vi "UI_Users_Manage.vi"() -> ()   [LabVIEW 2014]
panel:
  in  "选项卡控件":enum32{"添加用户", "删除用户"}(tab)
  in  "身份":u16(ring) items=["普通用户", "管理员"]
  in  "添加":bool
  in  "密码":string
  in  "添加用户名":string caption="用户名"
  in  "删除":bool
  in  "删除用户名":string caption="用户名"
  in  "导出excel":bool
  out "用户信息":string[][](table)
  in  "退出":bool
  # "用户管理"
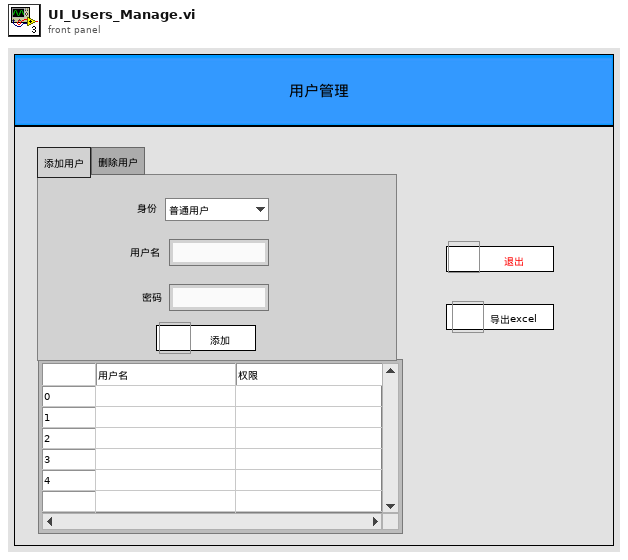
[diagram p1: front panel]
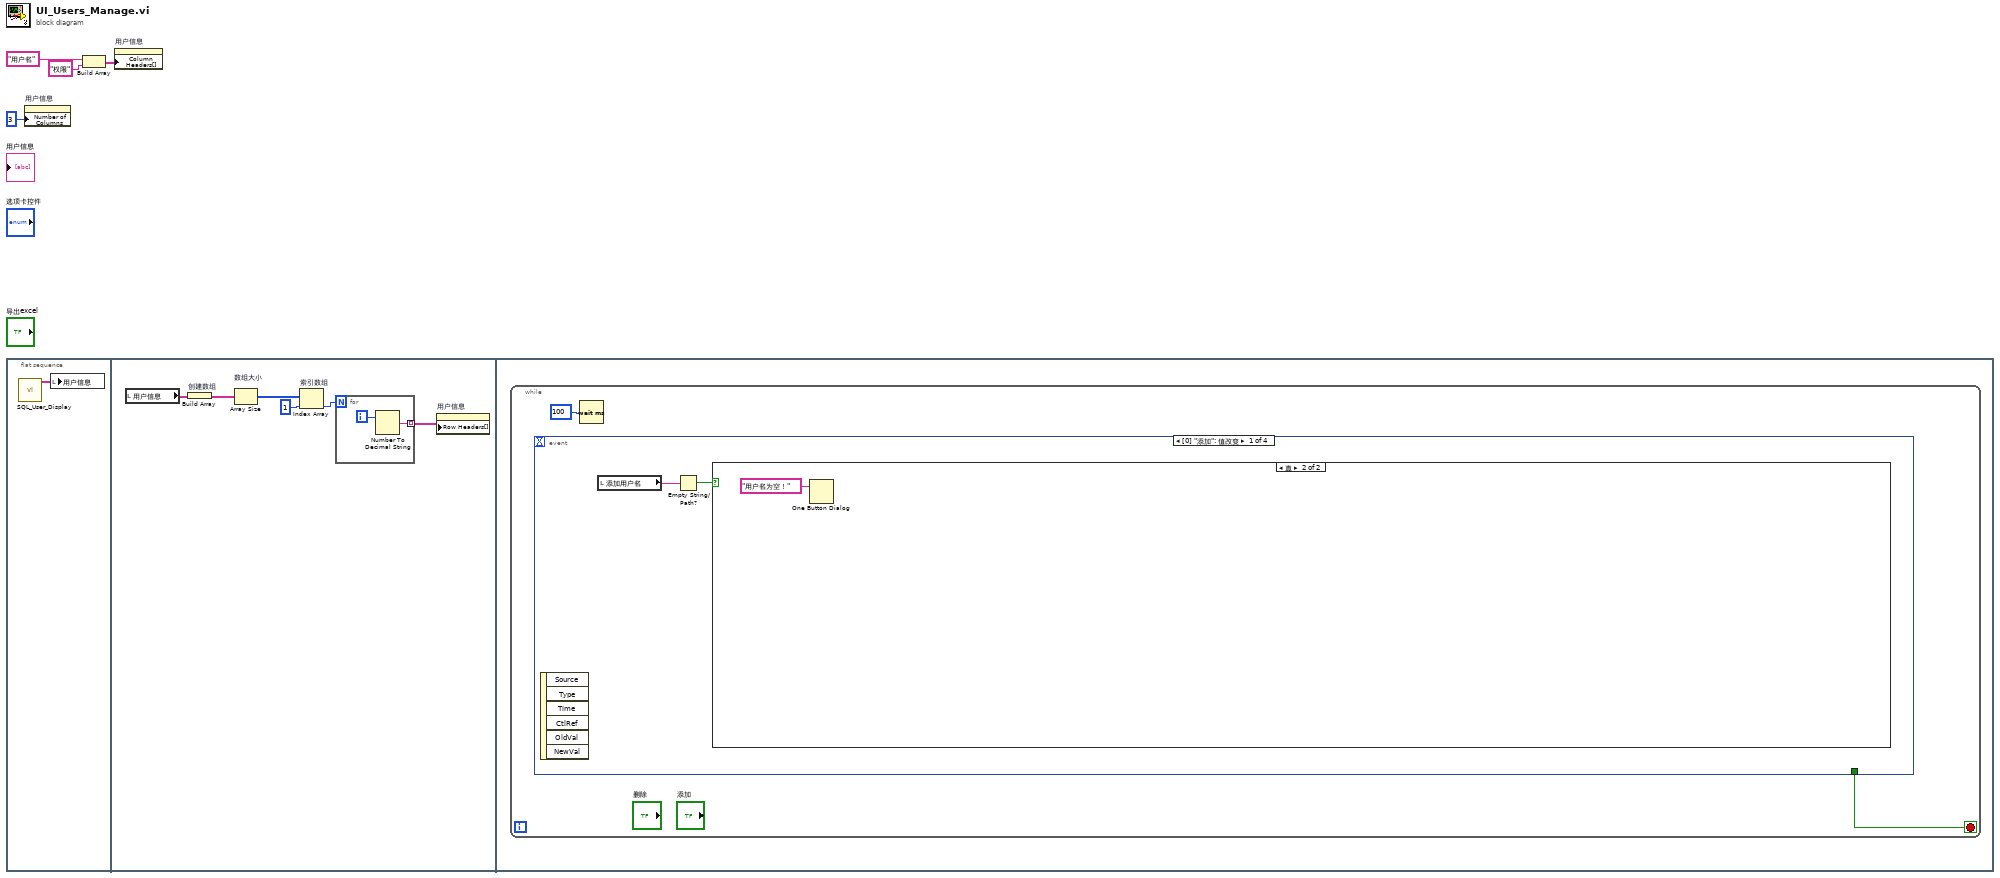
[diagram p0: block diagram]
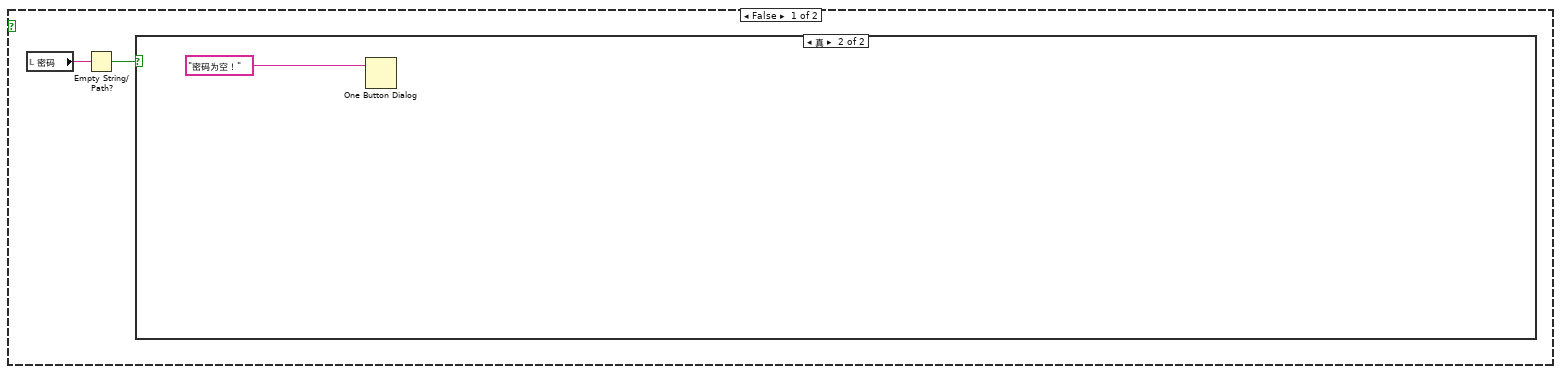
[diagram p2: hidden frame]
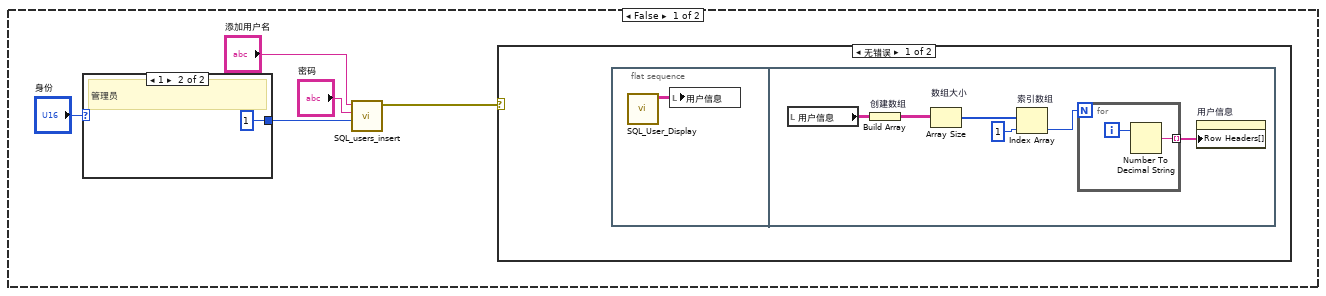
[diagram p3: hidden frame]
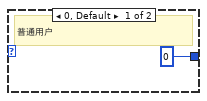
[diagram p5: hidden frame]
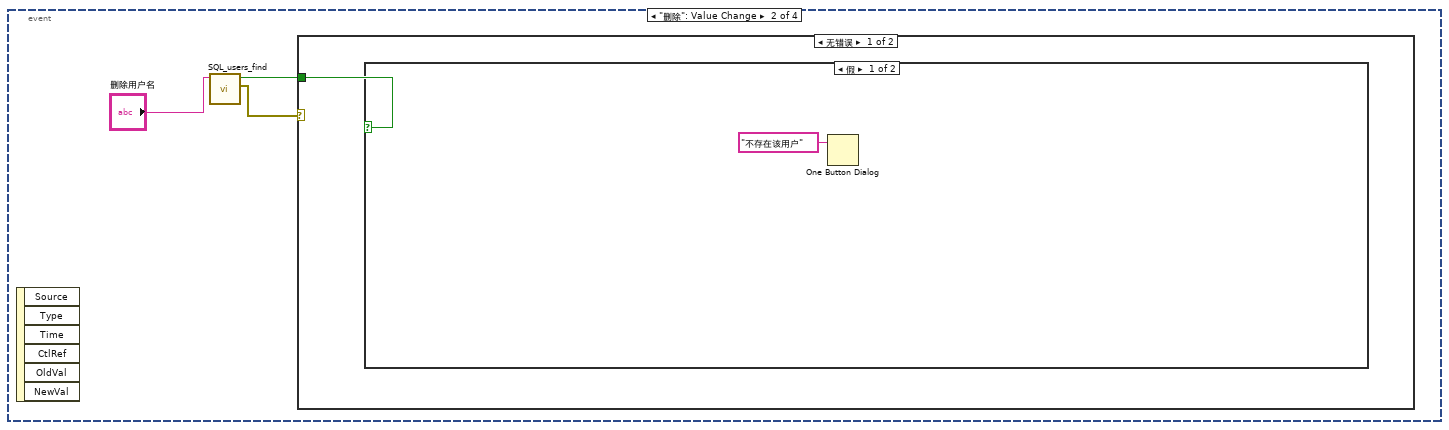
[diagram p6: hidden frame]
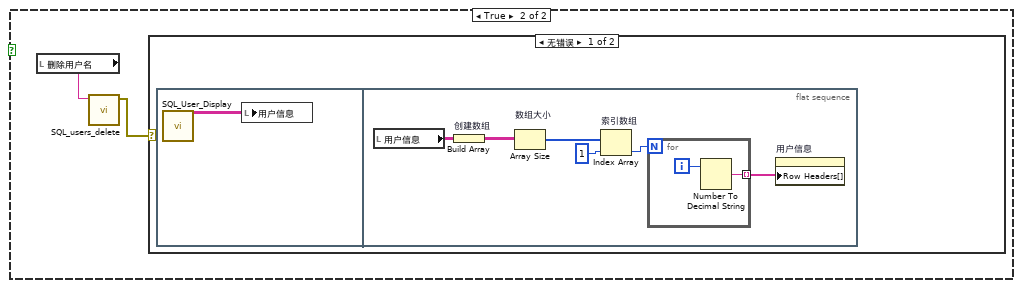
[diagram p7: hidden frame]
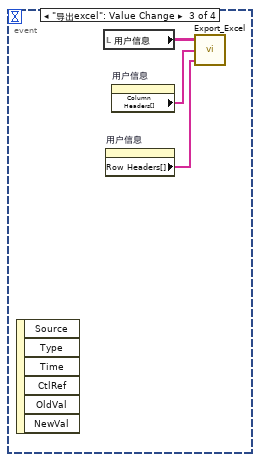
[diagram p10: hidden frame]
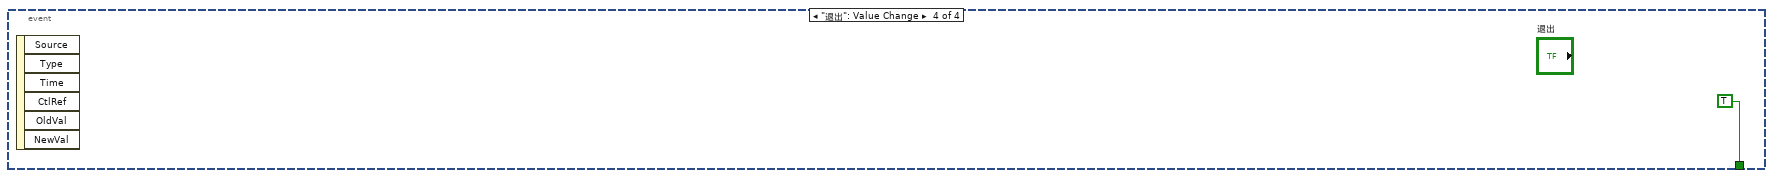
[diagram p11: hidden frame]
diagram:
  n1 = flat-sequence {
    frame #0 {
      n2 = call "SQL_User_Display.vi"() -> ("用户信息"=w5:string[][])  [unwired: 10 in]
      n3 = local write "用户信息"(w5) -> ()
    }
    frame #1 {
      n4 = local read "用户信息"() -> (w10:string[][])
      n5 = Build Array "创建数组"(w10) -> (w6:string[][][])
      n6 = Array Size "数组大小"(array=w6) -> (size(s)=w7:i32[])
      n7 = Index Array "索引数组"(array=w7, index=1) -> (element=w9:i32)
      n8 = for {
        N: w9 -> [_]
        tunnel: [w12] -> w11 mode=indexing
        i -> [w13]
        n9 = Number To Decimal String(number=w13) -> (decimal integer string=w12:string)  [unwired: 1 in]
      }
      n10 = property on="用户信息" class="Tbl (严格)"("Row Headers[]"=w11) -> ()  [unwired: 2 in, 2 out]
    }
    frame #2 {
      n11 = while {
        stop <- w14 stop-if-true
        n12 = event shown="[0] \"添加\": 值改变" {
          selector: _ -> [_ _ _ _]
          dyn-events: _ -> [_ _ _ _]
          timeout: _ -> [_ _ _ _]
          tunnel: [_ _ _ TRUE] -> w14
          event "添加": Value Change {
            n13 = event-data() -> ()  [unwired: 1 in, 6 out]
            n14 = local read "添加用户名"() -> (w16:string)
            n15 = Empty String/Path?(string/path=w16) -> (empty?=w17:bool)
            n16 = case shown="真" w17 {
              frame False {
                n17 = local read "密码"() -> (w18:string)
                n18 = Empty String/Path?(string/path=w18) -> (empty?=w19:bool)
                n19 = case shown="真" w19 {
                  frame False {
                    n20 = case shown="1" "身份" {
                      tunnel: [0 1] -> w24
                      frame 0, Default {
                        # "普通用户"
                      }
                      frame 1 {
                        # "管理员"
                      }
                    }
                    n21 = call "SQL_users_insert.vi"("权限"=w24, "密码"="密码", "用户名"="添加用户名") -> ("error out"=w20:errorcluster)  [unwired: 8 in]
                    n22 = case shown="无错误" w20 {
                      frame No Error {
                        n23 = flat-sequence {
                          frame #0 {
                            n24 = call "SQL_User_Display.vi"() -> ("用户信息"=w25:string[][])  [unwired: 10 in]
                            n25 = local write "用户信息"(w25) -> ()
                          }
                          frame #1 {
                            n26 = local read "用户信息"() -> (w27:string[][])
                            n27 = Build Array "创建数组"(w27) -> (w28:string[][][])
                            n28 = Array Size "数组大小"(array=w28) -> (size(s)=w29:i32[])
                            n29 = Index Array "索引数组"(array=w29, index=1) -> (element=w31:i32)
                            n30 = for {
                              N: w31 -> [_]
                              tunnel: [w32] -> w26 mode=indexing
                              i -> [w33]
                              n31 = Number To Decimal String(number=w33) -> (decimal integer string=w32:string)  [unwired: 1 in]
                            }
                            n32 = property on="用户信息" class="Tbl (严格)"("Row Headers[]"=w26) -> ()  [unwired: 2 in, 2 out]
                          }
                        }
                      }
                      frame Error {
                      }
                    }
                  }
                  frame True {
                    n33 = One Button Dialog(message="密码为空！" ("消息")) -> ()  [unwired: 1 in, 1 out]
                  }
                }
              }
              frame True {
                n34 = One Button Dialog(message="用户名为空！" ("消息")) -> ()  [unwired: 1 in, 1 out]
              }
            }
          }
          event "删除": Value Change {
            n35 = event-data() -> ()  [unwired: 1 in, 6 out]
            n36 = call "SQL_users_find.vi"("用户名"="删除用户名") -> ("error out"=w39:errorcluster, "是否存在该用户"=w38:bool)  [unwired: 9 in]
            n37 = case shown="无错误" w39 {
              tunnel: w38 -> [w41 _]
              frame No Error {
                n38 = case shown="假" w41 {
                  frame False {
                    n39 = One Button Dialog(message="不存在该用户" ("消息")) -> ()  [unwired: 1 in, 1 out]
                  }
                  frame True {
                    n40 = local read "删除用户名"() -> (w43:string)
                    n41 = call "SQL_users_delete.vi"("用户名"=w43) -> ("error out"=w44:errorcluster)  [unwired: 10 in]
                    n42 = case shown="无错误" w44 {
                      frame No Error {
                        n43 = flat-sequence {
                          frame #0 {
                            n44 = call "SQL_User_Display.vi"() -> ("用户信息"=w45:string[][])  [unwired: 10 in]
                            n45 = local write "用户信息"(w45) -> ()
                          }
                          frame #1 {
                            n46 = local read "用户信息"() -> (w47:string[][])
                            n47 = Build Array "创建数组"(w47) -> (w48:string[][][])
                            n48 = Array Size "数组大小"(array=w48) -> (size(s)=w49:i32[])
                            n49 = Index Array "索引数组"(array=w49, index=1) -> (element=w51:i32)
                            n50 = for {
                              N: w51 -> [_]
                              tunnel: [w52] -> w46 mode=indexing
                              i -> [w53]
                              n51 = Number To Decimal String(number=w53) -> (decimal integer string=w52:string)  [unwired: 1 in]
                            }
                            n52 = property on="用户信息" class="Tbl (严格)"("Row Headers[]"=w46) -> ()  [unwired: 2 in, 2 out]
                          }
                        }
                      }
                      frame Error {
                      }
                    }
                  }
                }
              }
              frame Error {
              }
            }
          }
          event "导出excel": Value Change {
            n53 = event-data() -> ()  [unwired: 1 in, 6 out]
            n54 = local read "用户信息"() -> (w54:string[][])
            n55 = property on="用户信息" class="Tbl (严格)"() -> ("Row Headers[]"=w55:string[])  [unwired: 2 in, 2 out]
            n56 = property on="用户信息" class="Tbl (严格)"() -> ("Column Headers[]"=w56:string[])  [unwired: 2 in, 2 out]
            n57 = call "Export_Excel.vi"("行首字符串[]"=w55, "列首字符串[]"=w56, "table"=w54) -> ()  [unwired: 1 in]
          }
          event "退出": Value Change {
            n58 = event-data() -> ()  [unwired: 1 in, 6 out]
          }
        }
        n59 = Wait (ms)(milliseconds to wait=u32 100 ("等待时间（毫秒）")) -> ()  [unwired: 1 out]
      }
    }
  }
  n60 = property on="用户信息" class="Tbl (严格)"("Number of Columns"=3) -> ()  [unwired: 2 in, 2 out]
  n61 = Build Array("用户名", "权限") -> (w1:string[])
  n62 = property on="用户信息" class="Tbl (严格)"("Column Headers[]"=w1) -> ()  [unwired: 2 in, 2 out]
